vi "Move abs mMc Edited.vi"(8 "error in (no error)":errorcluster, 9 "target pos in":dbl, 10 "Controller #":string, 11 "Port In":T1) -> (0 "error out":errorcluster, 3 "Port Out":T1)   [LabVIEW 2021]
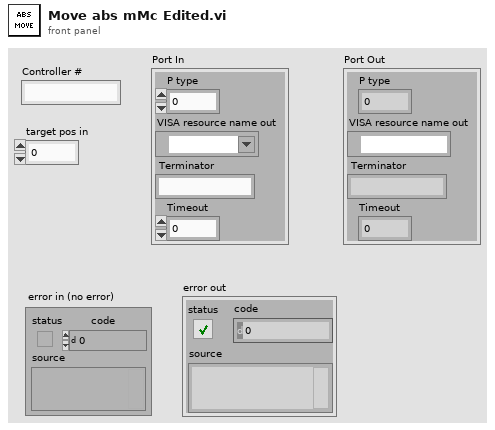
[diagram p1: front panel]
types:
  T1 = cluster{"P type":u16, "VISA resource name out":refnum<visa-resource-name>, " Terminator":string, "Timeout":i32}
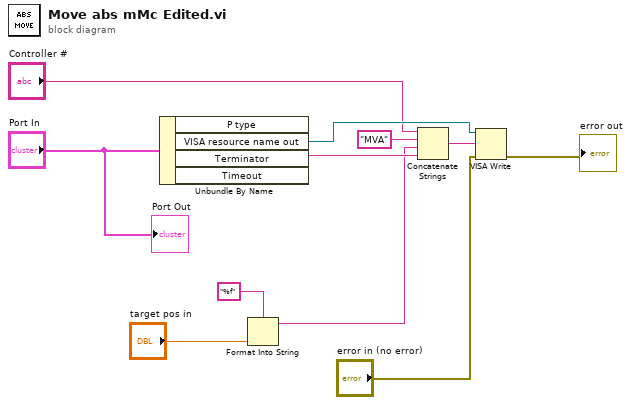
[diagram p0: block diagram]
diagram:
  n1 = Unbundle By Name("Port In") -> ("VISA resource name out"=w8:refnum<visa-resource-name>, "Terminator"=w5:string)  [unwired: 2 out]
  n2 = Format Into String(format string="%f", "target pos in") -> (resulting string=w4:string)  [unwired: 2 in, 1 out]
  n3 = Concatenate Strings("Controller #", "MVA" ("string"), w4, w5) -> (w10:string)
  n4 = VISA Write(VISA resource name=w8, write buffer=w10, error in (no error)="error in (no error)") -> (error out=→"error out":errorcluster)  [unwired: 2 out]
  "Port Out" <- "Port In"
